vi "InitializeOCUwriter.vi"(8 "error in (no error)":errorcluster, 11 "Boat Type":T1) -> (0 "error out":errorcluster, 3 "NetworkStreamWriter out":refnum<class "NetworkStreamWriter.lvclass">)   [LabVIEW 2013]
uses:
  RIO-OCU_Comm/NetworkStreams/Writer/NetworkStreamWriter.lvclass
  Data/TypeDefs/BoatType.ctl
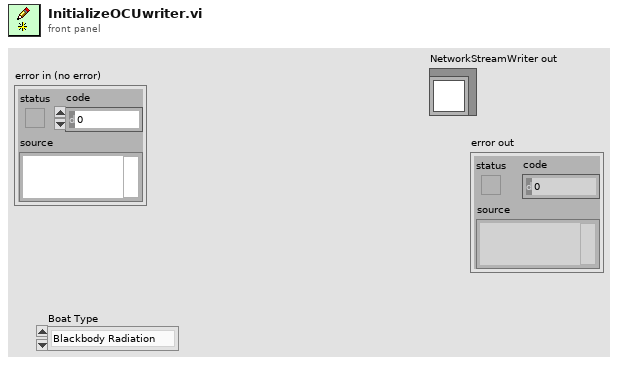
[diagram p1: front panel]
types:
  T1 = typedef "BoatType.ctl" = enum16{"Blackbody Radiation", "ReadLog", "Little boats", "Simulation", "Damn Yankee"}
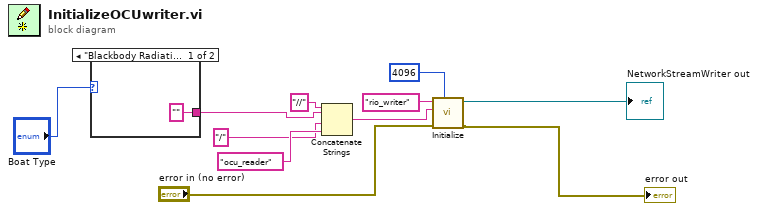
[diagram p0: block diagram]
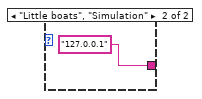
[diagram p2: hidden frame]
diagram:
  n1 = case shown="\"Blackbody Radiation\", Default" "Boat Type" {
    tunnel: ["" "127.0.0.1"] -> w2
    frame "Blackbody Radiation", Default {
    }
    frame "Little boats", "Simulation" {
    }
  }
  n2 = Concatenate Strings("//" ("string"), w2, "/", "ocu_reader" ("string")) -> (w5:string)
  n3 = call "Initialize.vi"("writer buffer size"=4096, "error in (no error)"="error in (no error)", "reader url"=w5, "writer name"="rio_writer") -> ("error out"=→"error out":errorcluster, "NetworkStreamWriter out"=→"NetworkStreamWriter out":refnum<class "NetworkStreamWriter.lvclass">)  [unwired: 6 in]
